vi "TEST_SPEECH.vi"() -> ()   [LabVIEW 2019]
uses:
  System.Speech
panel:
  in  "stop":bool
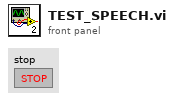
[diagram p1: front panel]
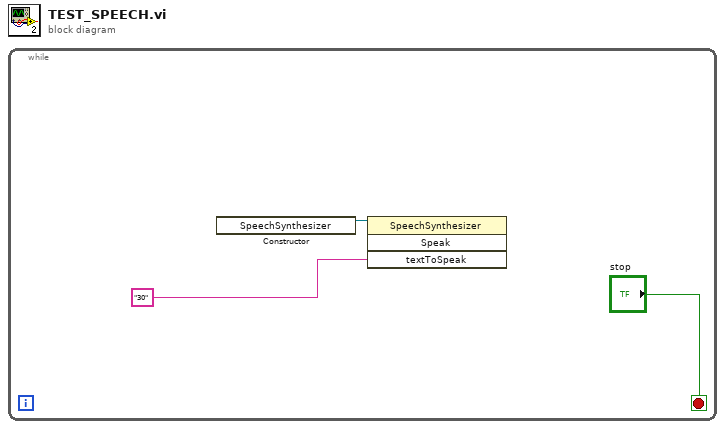
[diagram p0: block diagram]
diagram:
  n1 = while {
    stop <- "stop" stop-if-true
    n2 = constructor class="SpeechSynthesizer"() -> (reference out=w3:refnum<k24>)  [unwired: 3 in, 2 out]
    n3 = invoke class="SpeechSynthesizer" method="Speak"(reference=w3, "textToSpeak"="30") -> ()  [unwired: 2 in, 4 out]
  }
